vi "R_VG.vi"() -> ()   [LabVIEW 2020]
panel:
  in  "R > R-1?":dbl
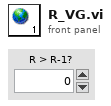
[diagram p1: front panel]
diagram:
